vi "CTRE_PigeonIMU_SetFusedHeading.vi"(8 "error in (no error)":errorcluster, 9 "TareType (SetValue)":T1 items=["SetValue"=0, "AddOffset"=1, "MatchCompass"=2, "SetOffset"=255], 10 "Value":dbl, 11 "PigeonIMUDevRef 2":T2={"DeviceStatus"={"status"=FALSE, "code"=0, "source"=""}, "Device Number"=0, "Type"=352321536, "Device ID"=0, "Handle"=0, "UsageFrame"=0, "Library Path"=path ""} {"Type" items=["CAN"=352321536, "TalonSRX"=33554432]}) -> (0 "error out":errorcluster, 3 "PigeonIMUDevRef":T2={"DeviceStatus"={"status"=FALSE, "code"=0, "source"=""}, "Device Number"=0, "Type"=352321536, "Device ID"=0, "Handle"=0, "UsageFrame"=0, "Library Path"=path ""} {"Type" items=["CAN"=352321536, "TalonSRX"=33554432]})   [LabVIEW 2016]
uses:
  CTRE_PigeonIMU_DeviceRef.ctl
  CTRE_PigeonIMU_ConnectionType.ctl
  CTRE_PigeonIMU_TareType.ctl
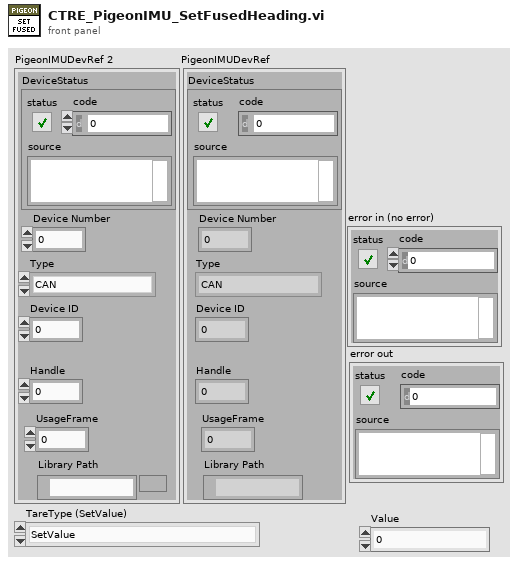
[diagram p1: front panel]
types:
  T1 = typedef "CTRE_PigeonIMU_TareType.ctl" = u8
  T2 = typedef "CTRE_PigeonIMU_DeviceRef.ctl" = cluster{"DeviceStatus":errorcluster, "Device Number":u8, "Type":T3, "Device ID":u32, "Handle":u64, "UsageFrame":u32, "Library Path":path}
  T3 = typedef "CTRE_PigeonIMU_ConnectionType.ctl" = u32
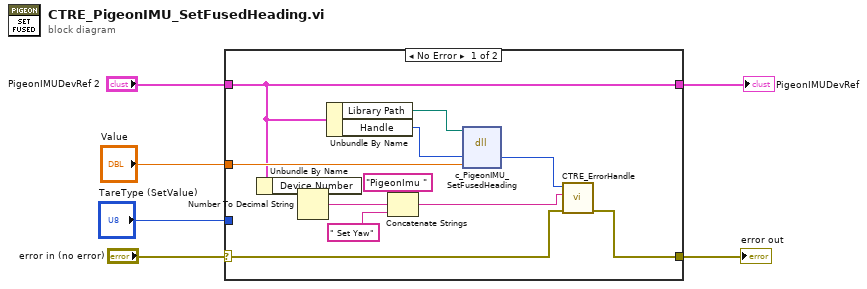
[diagram p0: block diagram]
diagram:
  n1 = case shown="No Error" "error in (no error)" {
    selector: "error in (no error)" -> [w9 w19]
    tunnel: [w10 w19] -> w5
    tunnel: [w7 w20] -> w3
    tunnel: "PigeonIMUDevRef 2" -> [w7 w20]
    tunnel: "Value" -> [w8 _]
    tunnel: "TareType (SetValue)" -> [_ _]
    frame No Error {
      n2 = Unbundle By Name(w7) -> ("Device Number"=w13:u8)
      n3 = Number To Decimal String(number=w13) -> (decimal integer string=w14:string)  [unwired: 1 in]
      n4 = Unbundle By Name(w7) -> ("Library Path"=w18:path, "Handle"=w17:u64)
      n5 = Concatenate Strings("PigeonImu " ("string"), w14, " Set Yaw" ("string")) -> (w11:string)
      n6 = dll-call lib="?" fn="c_PigeonIMU_SetFusedHeading"(path in=w18, "handle"=w17, "angleDeg"=w8) -> ("return type"=w12:i32)  [unwired: 4 in, 2 out]
      n7 = call "CTRE_ErrorHandle.vi"("error in"=w9, "origin"=w11, "code"=w12) -> ("error out"=w10:errorcluster)  [unwired: 8 in]
    }
    frame Error {
    }
  }
  "PigeonIMUDevRef" <- w3
  "error out" <- w5
